vi "WEBDAV Test.vi"() -> ()   [LabVIEW 2021]
uses:
  <vilib>/WebDAVClient/Advanced/FileInfo.ctl
  <vilib>/WebDAVClient/Simple Get File.vi
  <vilib>/WebDAVClient/NI_WebDAV.lvlib
panel:
  out "Time Stamp":timestamp
  out "uri":string
  out "file list":T1[](array[typedef])
  in  "Target IP":string
  in  "Folder name":path=path "C:/Users/KavinGovindaraj/Documents/TDMS"
  out "result string":string
  out "date/time string":string
  out "error out":errorcluster
  out "directory list":T1[](array[typedef])
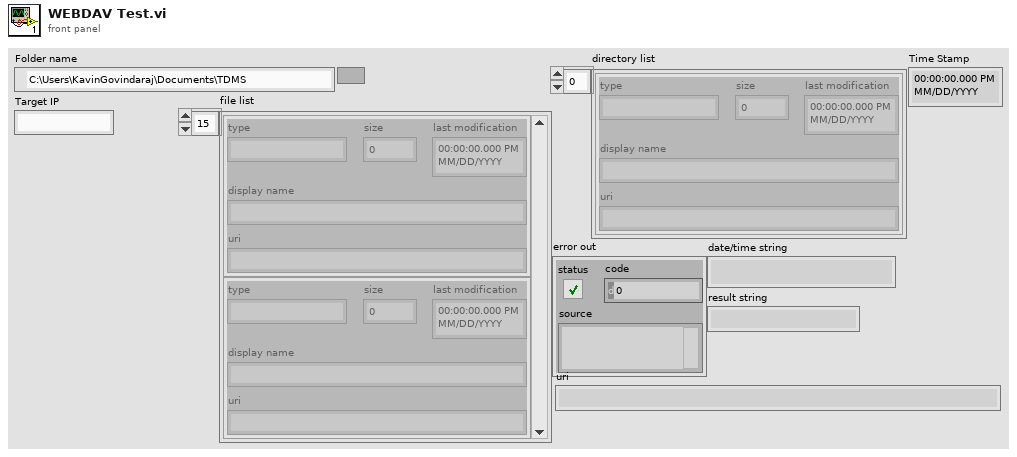
[diagram p1: front panel]
types:
  T1 = typedef "NI_WebDAV.lvlib/FileInfo.ctl" = cluster{"type":string, "size":u64, "last modification":timestamp, "display name":string, "uri":string}
  T2 = typedef "NI_WebDAV.lvlib/SessionHandle.ctl" = refnum<k1>
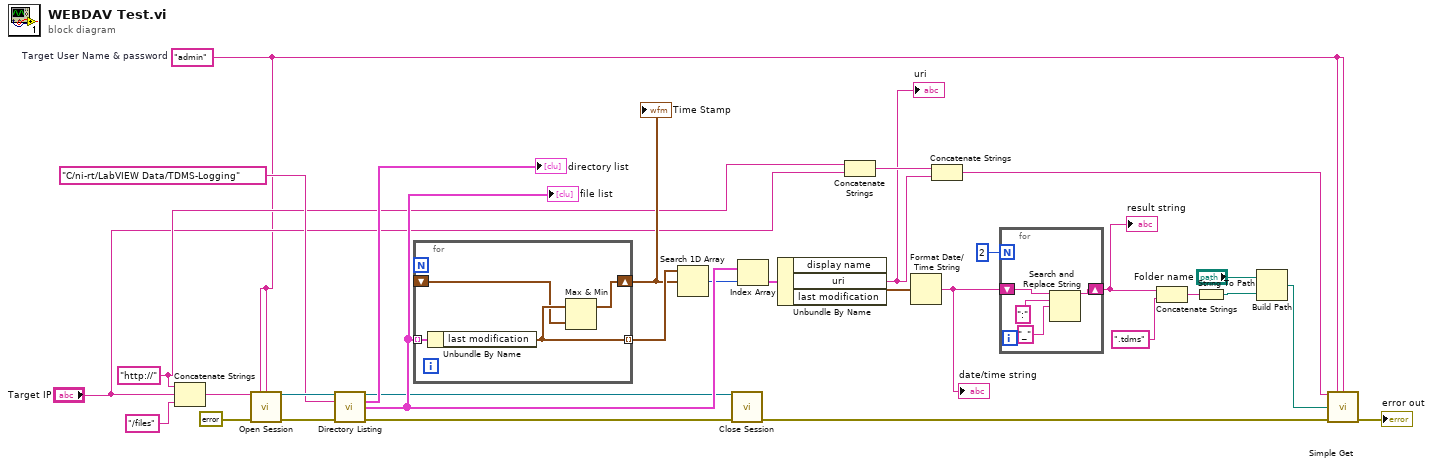
[diagram p0: block diagram]
diagram:
  w7 = "http://" ("remote file uri")
  w1 = "admin"  # Target User Name & password
  n1 = Concatenate Strings(w7, "Target IP", "/files" ("remote file uri")) -> (w8:string)
  n2 = call <vilib>:"Open Session.vi"("host uri prefix"=w8, "username"=w1, "password"=w1, "error in (no error)"=errorcluster {"status"=FALSE, "code"=0, "source"=""}) -> ("session handle out"=w31:T2, "error out"=w29:errorcluster)  [unwired: 10 in]
  n3 = call <vilib>:"Directory Listing.vi"("session handle"=w31, "relative uri"="C/ni-rt/LabVIEW Data/TDMS-Logging", "error in (no error)"=w29) -> ("session handle out"=w4:T2, "directory list"=→"directory list":T1[], "file list"=w24:T1[], "error out"=w3:errorcluster)  [unwired: 9 in]
  "file list" <- w24
  n4 = for {
    tunnel: w24 -> [w35] mode=indexing
    tunnel: [w34] -> w26 mode=indexing
    shift-right: [w33] -> w25
    shift-left: _ -> [w32]
    n5 = Unbundle By Name(w35) -> ("last modification"=w34:timestamp)
    n6 = Max & Min(x=w34, y=w32) -> (max(x,y)=w33:timestamp)  [unwired: 1 out]
  }
  "Time Stamp" <- w25
  n7 = Search 1D Array(1D array=w26, element=w25) -> (index of element=w23:i32)  [unwired: 1 in]
  n8 = call <vilib>:"Close Session.vi"("session handle"=w4, "error in (no error)"=w3) -> ("error out"=w21:errorcluster)  [unwired: 13 in]
  n9 = Index Array(array=w24, index=w23) -> (element=w22:T1)
  n10 = Unbundle By Name(w22) -> ("uri"=w2:string, "last modification"=w17:timestamp)  [unwired: 1 out]
  "uri" <- w2
  n11 = Concatenate Strings(w7, "Target IP") -> (w5:string)
  n12 = Format Date/Time String(seconds (now)=w17) -> (date/time string=w12:string)  [unwired: 2 in]
  "date/time string" <- w12
  n13 = Concatenate Strings(w5, w2) -> (w19:string)
  n14 = for {
    N: 2 -> [_]
    shift-right: [w37] -> w11
    shift-left: w12 -> [w39]
    n15 = Search and Replace String(input string=w39, search string=":", replace string="_" ("replace string (\"\")")) -> (result string=w37:string)  [unwired: 5 in, 3 out]
  }
  "result string" <- w11
  n16 = Concatenate Strings(w11, ".tdms" ("string")) -> (w15:string)
  n17 = String To Path(string=w15) -> (path=w14:path)
  n18 = Build Path(base path="Folder name", name or relative path=w14) -> (appended path=w18:path)
  n19 = call-poly <vilib>:"Simple Get.vi"("remote file uri"=w19, "username"=w1, "password"=w1, "local file path"=w18, "error in (no error)"=w21) -> ("error out"=→"error out":errorcluster)  [unwired: 9 in, 1 out]
